vi "Filter Table String.vi"() -> ()   [LabVIEW 2010]
panel:
  in  "input string":string
  out "array":dbl[][](array[numeric])
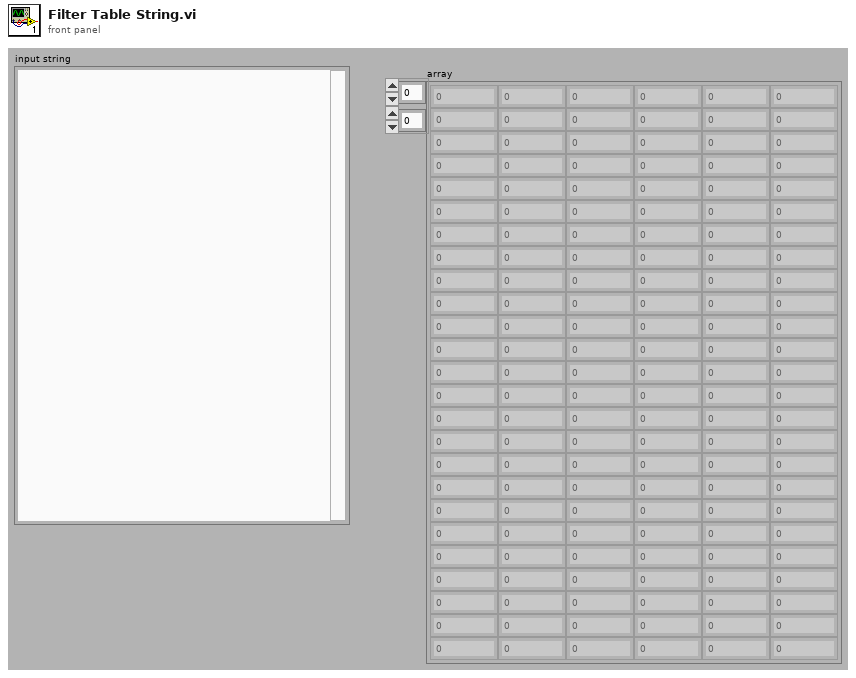
[diagram p1: front panel]
diagram:
  w2 = TRUE ("replace all? (F)")
  (unwired) "N,VBAT Voltage,VBAT Current,DVDD Current,Loaded DVDD Voltage,Loaded DVDD Ripple"
  (unwired) "0.000E+0, 4.199E+0, 20.109E-3, -19.994E-3, 2.448E+0, 109.310E-3 1.000E+0, 4.189E+0, 20.108E-3, -19.994E-3, 2.448E+0, 133.222E-3 2.000E+0, 4.179E+0, 20.108E-3, -19.994E-3, 2.448E+0, 109.310E-3 3.000E+0, 4.169E+0, 20.108E-3, -19.994E-3, 2.449E+0, 126.390E-3 4.000E+0, 4.159E+0, 20.108E-3, -19.994E-3, 2.448E+0, 119.558E-3 5.000E+0, 4.149E+0, 20.107E-3, -19.994E-3, 2.448E+0, 153.717E-3 6.000E+0, 4.139E+0, 20.107E-3, -19.994E-3, 2.448E+0, 122.974E-3 7.000E+0, 4.129E+0, 20.107E-3, -19.994E-3, 2.448E+0, 126.390E-3 8.000E+0, 4.119E+0, 20.107E-3, -19.994E-3, 2.448E+0, 109.310E-3 9.000E+0, 4.109E+0, 20.106E-3, -19.994E-3, 2.448E+0, 112.726E-3 10.000E+0, 4.099E+0, 20.106E-3, -19.994E-3, 2.448E+0, 116.142E-3 11.000E+0, 4.089E+0, 20.106E-3, -19.994E-3, 2.448E+0, 126.390E-3 12.000E+0, 4.079E+0, 20.106E-3, -19.994E-3, 2.448E+0, 122.974E-3 13.000E+0, 4.069E+0, 20.106E-3, -19.994E-3, 2.448E+0, 129.806E-3 14.000E+0, 4.059E+0, 20.106E-3, -19.994E-3, 2.448E+0, 116.142E-3 15.000E+0, 4.049E+0, 20.105E-3, -19.994E-3, 2.448E+0, 119.558E-3 16.000E+0, 4.039E+0, 20.105E-3, -19.994E-3, 2.448E+0, 116.142E-3 17.000E+0, 4.029E+0, 20.105E-3, -19.994E-3, 2.448E+0, 119.558E-3 18.000E+0, 4.019E+0, 20.105E-3, -19.994E-3, 2.448E+0, 105.894E-3 19.000E+0, 4.009E+0, 20.104E-3, -19.994E-3, 2.448E+0, 105.894E-3 20.000E+0, 3.999E+0, 20.104E-3, -19.994E-3, 2.448E+0, 126.390E-3 21.000E+0, 3.989E+0, 20.104E-3, -19.994E-3, 2.448E+0, 105.894E-3 22.000E+0, 3.979E+0, 20.104E-3, -19.994E-3, 2.448E+0, 143.469E-3 23.000E+0, 3.969E+0, 20.103E-3, -19.994E-3, 2.448E+0, 112.726E-3 24.000E+0, 3.959E+0, 20.103E-3, -19.994E-3, 2.448E+0, 112.726E-3 25.000E+0, 3.949E+0, 20.103E-3, -19.994E-3, 2.448E+0, 126.390E-3 26.000E+0, 3.939E+0, 20.103E-3, -19.994E-3, 2.448E+0, 122.974E-3 27.000E+0, 3.929E+0, 20.103E-3, -19.994E-3, 2.448E+0, 129.806E-3 28.000E+0, 3.919E+0, 20.103E-3, -19.994E-3, 2.448E+0, 126.390E-3 29.000E+0, 3.909E+0, 20.102E-3, -19.994E-3, 2.448E+0, 122.974E-3 30.000E+0, 3.899E+0, 20.102E-3, -19.994E-3, 2.448E+0, 129.806E-3 31.000E+0, 3.889E+0, 20.102E-3, -19.994E-3, 2.448E+0, 136.638E-3 32.000E+0, 3.879E+0, 20.102E-3, -19.994E-3, 2.448E+0, 140.053E-3 33.000E+0, 3.869E+0, 20.102E-3, -19.994E-3, 2.448E+0, 122.974E-3 34.000E+0, 3.859E+0, 20.101E-3, -19.994E-3, 2.448E+0, 105.894E-3 35.000E+0, 3.849E+0, 20.102E-3, -19.994E-3, 2.447E+0, 140.053E-3 36.000E+0, 3.839E+0, 20.101E-3, -19.994E-3, 2.448E+0, 119.558E-3 37.000E+0, 3.829E+0, 20.101E-3, -19.994E-3, 2.448E+0, 112.726E-3 38.000E+0, 3.819E+0, 20.101E-3, -19.994E-3, 2.447E+0, 122.974E-3 39.000E+0, 3.809E+0, 20.100E-3, -19.994E-3, 2.448E+0, 116.142E-3 40.000E+0, 3.799E+0, 20.101E-3, -19.994E-3, 2.448E+0, 133.222E-3 41.000E+0, 3.789E+0, 20.100E-3, -19.994E-3, 2.448E+0, 122.974E-3 42.000E+0, 3.779E+0, 20.100E-3, -19.994E-3, 2.448E+0, 126.390E-3 43.000E+0, 3.769E+0, 20.100E-3, -19.994E-3, 2.448E+0, 129.806E-3 44.000E+0, 3.759E+0, 20.100E-3, -19.994E-3, 2.447E+0, 112.726E-3 45.000E+0, 3.749E+0, 20.100E-3, -19.994E-3, 2.448E+0, 133.222E-3 46.000E+0, 3.739E+0, 20.099E-3, -19.994E-3, 2.448E+0, 112.726E-3 47.000E+0, 3.729E+0, 20.099E-3, -19.994E-3, 2.448E+0, 122.974E-3 48.000E+0, 3.719E+0, 20.099E-3, -19.994E-3, 2.448E+0, 133.222E-3 49.000E+0, 3.709E+0, 20.099E-3, -19.994E-3, 2.448E+0, 126.390E-3 50.000E+0, 3.699E+0, 20.098E-3, -19.994E-3, 2.447E+0, 112.726E-3 51.000E+0, 3.689E+0, 20.099E-3, -19.994E-3, 2.448E+0, 126.390E-3 52.000E+0, 3.679E+0, 20.098E-3, -19.994E-3, 2.447E+0, 105.894E-3 53.000E+0, 3.670E+0, 20.098E-3, -19.994E-3, 2.447E+0, 112.726E-3 54.000E+0, 3.659E+0, 20.098E-3, -19.994E-3, 2.447E+0, 122.974E-3 55.000E+0, 3.649E+0, 20.098E-3, -19.994E-3, 2.447E+0, 109.310E-3 56.000E+0, 3.639E+0, 20.098E-3, -19.994E-3, 2.447E+0, 95.646E-3 57.000E+0, 3.629E+0, 20.097E-3, -19.994E-3, 2.447E+0, 129.806E-3 58.000E+0, 3.620E+0, 20.097E-3, -19.994E-3, 2.447E+0, 99.062E-3 59.000E+0, 3.609E+0, 20.097E-3, -19.994E-3, 2.447E+0, 116.142E-3 60.000E+0, 3.599E+0, 20.097E-3, -19.994E-3, 2.447E+0, 143.469E-3 61.000E+0, 3.589E+0, 20.097E-3, -19.994E-3, 2.447E+0, 116.142E-3 62.000E+0, 3.579E+0, 20.097E-3, -19.994E-3, 2.447E+0, 112.726E-3 63.000E+0, 3.570E+0, 20.096E-3, -19.994E-3, 2.447E+0, 116.142E-3 64.000E+0, 3.559E+0, 20.096E-3, -19.994E-3, 2.447E+0, 122.974E-3 65.000E+0, 3.549E+0, 20.096E-3, -19.994E-3, 2.448E+0, 116.142E-3 66.000E+0, 3.539E+0, 20.096E-3, -19.994E-3, 2.447E+0, 140.053E-3 67.000E+0, 3.530E+0, 20.095E-3, -19.994E-3, 2.447E+0, 122.974E-3 68.000E+0, 3.520E+0, 20.096E-3, -19.994E-3, 2.447E+0, 112.726E-3 69.000E+0, 3.509E+0, 20.095E-3, -19.994E-3, 2.447E+0, 116.142E-3 70.000E+0, 3.499E+0, 20.095E-3, -19.994E-3, 2.447E+0, 126.390E-3 71.000E+0, 3.490E+0, 20.095E-3, -19.994E-3, 2.447E+0, 119.558E-3 72.000E+0, 3.480E+0, 20.095E-3, -19.994E-3, 2.447E+0, 105.894E-3 73.000E+0, 3.470E+0, 20.095E-3, -19.994E-3, 2.447E+0, 105.894E-3 74.000E+0, 3.459E+0, 20.095E-3, -19.994E-3, 2.447E+0, 122.974E-3 75.000E+0, 3.449E+0, 20.095E-3, -19.994E-3, 2.447E+0, 133.222E-3 76.000E+0, 3.440E+0, 20.094E-3, -19.994E-3, 2.447E+0, 105.894E-3 77.000E+0, 3.430E+0, 20.094E-3, -19.994E-3, 2.447E+0, 116.142E-3 78.000E+0, 3.420E+0, 20.094E-3, -19.994E-3, 2.447E+0, 122.974E-3 79.000E+0, 3.410E+0, 20.093E-3, -19.994E-3, 2.447E+0, 116.142E-3 80.000E+0, 3.400E+0, 20.093E-3, -19.994E-3, 2.447E+0, 119.558E-3 81.000E+0, 3.390E+0, 20.093E-3, -19.994E-3, 2.447E+0, 109.310E-3 82.000E+0, 3.380E+0, 20.093E-3, -19.994E-3, 2.448E+0, 129.806E-3 83.000E+0, 3.370E+0, 20.093E-3, -19.994E-3, 2.447E+0, 122.974E-3 84.000E+0, 3.360E+0, 20.093E-3, -19.994E-3, 2.447E+0, 122.974E-3 85.000E+0, 3.350E+0, 20.093E-3, -19.994E-3, 2.447E+0, 153.717E-3 86.000E+0, 3.340E+0, 20.093E-3, -19.994E-3, 2.447E+0, 122.974E-3 87.000E+0, 3.330E+0, 20.092E-3, -19.994E-3, 2.447E+0, 119.558E-3 88.000E+0, 3.320E+0, 20.092E-3, -19.994E-3, 2.447E+0, 126.390E-3 89.000E+0, 3.310E+0, 20.092E-3, -19.994E-3, 2.447E+0, 133.222E-3 90.000E+0, 3.300E+0, 20.092E-3, -19.994E-3, 2.447E+0, 133.222E-3 91.000E+0, 3.290E+0, 20.092E-3, -19.994E-3, 2.447E+0, 136.638E-3 92.000E+0, 3.280E+0, 20.092E-3, -19.994E-3, 2.447E+0, 126.390E-3 93.000E+0, 3.270E+0, 20.091E-3, -19.994E-3, 2.447E+0, 133.222E-3 94.000E+0, 3.260E+0, 20.091E-3, -19.994E-3, 2.447E+0, 119.558E-3 95.000E+0, 3.250E+0, 20.092E-3, -19.994E-3, 2.447E+0, 133.222E-3 96.000E+0, 3.240E+0, 20.091E-3, -19.994E-3, 2.447E+0, 119.558E-3 97.000E+0, 3.230E+0, 20.091E-3, -19.994E-3, 2.447E+0, 105.894E-3 98.000E+0, 3.220E+0, 20.091E-3, -19.994E-3, 2.447E+0, 119.558E-3 99.000E+0, 3.210E+0, 20.090E-3, -19.994E-3, 2.447E+0, 136.638E-3 100.000E+0, 3.200E+0, 20.090E-3, -19.994E-3, 2.446E+0, 133.222E-3 101.000E+0, 3.190E+0, 20.090E-3, -19.994E-3, 2.446E+0, 112.726E-3 102.000E+0, 3.180E+0, 20.090E-3, -19.994E-3, 2.446E+0, 126.390E-3 103.000E+0, 3.170E+0, 20.090E-3, -19.994E-3, 2.446E+0, 126.390E-3 104.000E+0, 3.160E+0, 20.090E-3, -19.994E-3, 2.446E+0, 133.222E-3 105.000E+0, 3.150E+0, 20.090E-3, -19.994E-3, 2.446E+0, 119.558E-3 106.000E+0, 3.140E+0, 20.090E-3, -19.994E-3, 2.446E+0, 112.726E-3 107.000E+0, 3.130E+0, 20.090E-3, -19.994E-3, 2.446E+0, 116.142E-3 108.000E+0, 3.120E+0, 20.089E-3, -19.994E-3, 2.446E+0, 153.717E-3 109.000E+0, 3.110E+0, 20.090E-3, -19.994E-3, 2.446E+0, 126.390E-3 110.000E+0, 3.100E+0, 20.089E-3, -19.994E-3, 2.445E+0, 109.310E-3 111.000E+0, 3.090E+0, 20.089E-3, -19.994E-3, 2.446E+0, 109.310E-3 112.000E+0, 3.080E+0, 20.089E-3, -19.994E-3, 2.446E+0, 109.310E-3 113.000E+0, 3.070E+0, 20.089E-3, -19.994E-3, 2.446E+0, 122.974E-3 114.000E+0, 3.060E+0, 20.089E-3, -19.994E-3, 2.446E+0, 122.974E-3 115.000E+0, 3.050E+0, 20.088E-3, -19.994E-3, 2.446E+0, 116.142E-3 116.000E+0, 3.040E+0, 20.088E-3, -19.994E-3, 2.446E+0, 112.726E-3 117.000E+0, 3.030E+0, 20.088E-3, -19.994E-3, 2.446E+0, 119.558E-3 118.000E+0, 3.020E+0, 20.088E-3, -19.994E-3, 2.446E+0, 136.638E-3 119.000E+0, 3.010E+0, 20.088E-3, -19.994E-3, 2.445E+0, 122.974E-3 120.000E+0, 3.000E+0, 20.088E-3, -19.994E-3, 2.445E+0, 112.726E-3 121.000E+0, 2.990E+0, 20.087E-3, -19.994E-3, 2.446E+0, 140.053E-3 122.000E+0, 2.980E+0, 20.087E-3, -19.994E-3, 2.446E+0, 133.222E-3 123.000E+0, 2.970E+0, 20.088E-3, -19.994E-3, 2.446E+0, 126.390E-3 124.000E+0, 2.960E+0, 20.087E-3, -19.994E-3, 2.446E+0, 122.974E-3 125.000E+0, 2.950E+0, 20.087E-3, -19.994E-3, 2.445E+0, 133.222E-3 126.000E+0, 2.940E+0, 20.087E-3, -19.994E-3, 2.445E+0, 119.558E-3 127.000E+0, 2.930E+0, 20.087E-3, -19.994E-3, 2.444E+0, 129.806E-3 128.000E+0, 2.920E+0, 20.087E-3, -19.994E-3, 2.445E+0, 129.806E-3 129.000E+0, 2.910E+0, 20.086E-3, -19.994E-3, 2.444E+0, 116.142E-3 130.000E+0, 2.900E+0, 20.086E-3, -19.994E-3, 2.445E+0, 112.726E-3 131.000E+0, 2.890E+0, 20.086E-3, -19.994E-3, 2.444E+0, 105.894E-3 132.000E+0, 2.880E+0, 20.087E-3, -19.994E-3, 2.444E+0, 109.310E-3 133.000E+0, 2.870E+0, 20.087E-3, -19.994E-3, 2.443E+0, 112.726E-3 134.000E+0, 2.860E+0, 20.086E-3, -19.994E-3, 2.443E+0, 105.894E-3 135.000E+0, 2.850E+0, 20.086E-3, -19.994E-3, 2.443E+0, 122.974E-3 136.000E+0, 2.840E+0, 20.086E-3, -19.994E-3, 2.443E+0, 112.726E-3 137.000E+0, 2.830E+0, 20.086E-3, -19.994E-3, 2.442E+0, 122.974E-3 138.000E+0, 2.820E+0, 20.085E-3, -19.994E-3, 2.442E+0, 122.974E-3 139.000E+0, 2.810E+0, 20.085E-3, -19.994E-3, 2.440E+0, 112.726E-3 140.000E+0, 2.800E+0, 20.086E-3, -19.994E-3, 2.440E+0, 126.390E-3 141.000E+0, 2.790E+0, 20.085E-3, -19.994E-3, 2.439E+0, 119.558E-3 142.000E+0, 2.780E+0, 20.086E-3, -19.994E-3, 2.437E+0, 119.558E-3 143.000E+0, 2.770E+0, 20.085E-3, -19.994E-3, 2.435E+0, 129.806E-3 144.000E+0, 2.760E+0, 20.085E-3, -19.994E-3, 2.431E+0, 119.558E-3 145.000E+0, 2.750E+0, 20.084E-3, -19.994E-3, 2.424E+0, 129.806E-3 146.000E+0, 2.740E+0, 20.084E-3, -19.994E-3, 2.414E+0, 146.885E-3 147.000E+0, 2.730E+0, 20.084E-3, -19.994E-3, 2.404E+0, 116.142E-3 148.000E+0, 2.720E+0, 20.083E-3, -19.994E-3, 2.393E+0, 112.726E-3 149.000E+0, 2.710E+0, 20.083E-3, -19.994E-3, 2.383E+0, 116.142E-3 150.000E+0, 2.700E+0, 20.083E-3, -19.994E-3, 2.373E+0, 116.142E-3 151.000E+0, 2.690E+0, 20.082E-3, -19.994E-3, 2.363E+0, 133.222E-3 152.000E+0, 2.680E+0, 20.082E-3, -19.994E-3, 2.353E+0, 136.638E-3 153.000E+0, 2.670E+0, 20.082E-3, -19.994E-3, 2.343E+0, 129.806E-3 154.000E+0, 2.660E+0, 20.082E-3, -19.994E-3, 2.332E+0, 122.974E-3 155.000E+0, 2.650E+0, 20.081E-3, -19.994E-3, 2.323E+0, 126.390E-3 156.000E+0, 2.640E+0, 20.081E-3, -19.994E-3, 2.312E+0, 133.222E-3 157.000E+0, 2.630E+0, 20.081E-3, -19.994E-3, 2.302E+0, 126.390E-3 158.000E+0, 2.620E+0, 20.080E-3, -19.994E-3, 2.291E+0, 129.806E-3 159.000E+0, 2.610E+0, 20.080E-3, -19.994E-3, 2.281E+0, 133.222E-3 160.000E+0, 2.600E+0, 20.080E-3, -19.994E-3, 2.270E+0, 146.885E-3 161.000E+0, 2.590E+0, 20.079E-3, -19.994E-3, 2.260E+0, 109.310E-3 162.000E+0, 2.580E+0, 20.079E-3, -19.994E-3, 2.249E+0, 140.053E-3 163.000E+0, 2.570E+0, 20.079E-3, -19.994E-3, 2.239E+0, 109.310E-3 164.000E+0, 2.560E+0, 20.078E-3, -19.994E-3, 2.228E+0, 109.310E-3 165.000E+0, 2.550E+0, 20.078E-3, -19.994E-3, 2.219E+0, 119.558E-3 166.000E+0, 2.540E+0, 20.078E-3, -19.994E-3, 2.207E+0, 140.053E-3 167.000E+0, 2.530E+0, 20.077E-3, -19.994E-3, 2.198E+0, 112.726E-3 168.000E+0, 2.520E+0, 20.077E-3, -19.994E-3, 2.187E+0, 140.053E-3 169.000E+0, 2.510E+0, 20.077E-3, -19.994E-3, 2.176E+0, 109.310E-3 170.000E+0, 2.500E+0, 20.076E-3, -19.994E-3, 2.165E+0, 136.638E-3 "
  n1 = Search and Replace String(replace all?=w2, input string="input string", search string=", ", replace string="\t") -> (result string=w8:string)  [unwired: 4 in, 3 out]
  n2 = Search and Replace String(replace all?=w2, input string=w8, search string=" ", replace string="\r\n") -> (result string=w5:string)  [unwired: 4 in, 3 out]
  n3 = Spreadsheet String To Array(format string="%f", spreadsheet string=w5) -> (array=→"array":dbl[][])  [unwired: 2 in]
